vi "RT.vi"() -> ()   [LabVIEW 2023]
uses:
  <vilib>/FPGAPlugInAG/cRIO-9055/niLvFpga_Open_cRIO-9055.vi
  <vilib>/Utility/error.llb/Error Cluster From Error Code.vi
  <vilib>/rvi/errors/niLvFpgaAdjustHostInterfaceError.vi
  <vilib>/FPGAPlugInAG/cRIO-9055/niLvFpga_Run_cRIO-9055.vi
  <vilib>/FPGAPlugInAG/cRIO-9055/niLvFpga_Close_cRIO-9055.vi
  <vilib>/rvi/interface/nirviOpenFPGA/nirviOpenFPGA.xnode
  FPGA Bitfiles/projectni_FPGATarget_FPGA_GhjuFY+lihg.lvbitx
  Basic Logging/FPGA/FPGA.vi
  <vilib>/rvi/interface/nirviMethod/nirviMethod.xnode
  <vilib>/rvi/interface/nirviReadWriteControl/nirviReadWriteControl.xnode
  <vilib>/rvi/interface/nirviCloseFPGA/nirviCloseFPGA.xnode
  <vilib>/rvi/errors/niLvFpgaMergeErrorWithErrorCode.vi
  <vilib>/FPGAPlugInAG/cRIO-9055/niLvFpga_StartFifo_cRIO-9055.vi
  NiFpgaLv.dll
  <vilib>/FPGAPlugInAG/cRIO-9055/niLvFpga_ReadFifo_cRIO-9055.vi
panel:
  out "error out":errorcluster
  out "Timed Out?":bool
  out "Analog Input Chart":dbl[][](graph)
  in  "stop":bool
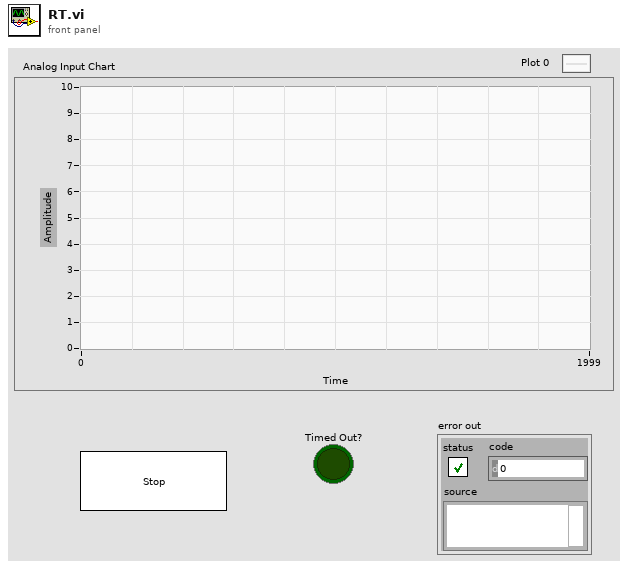
[diagram p1: front panel]
types:
  T1 = enum16{"open", "open or create", "create or replace", "create", "open (read-only)"}
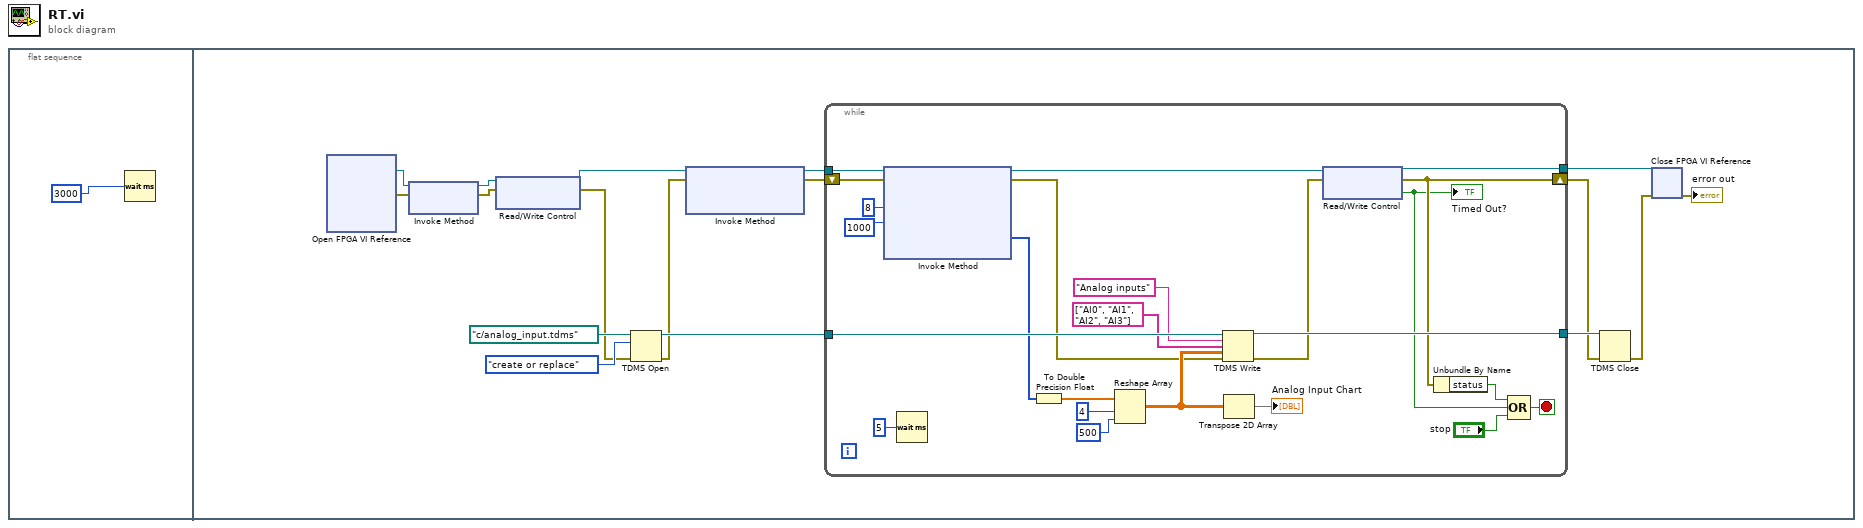
[diagram p0: block diagram]
diagram:
  n1 = flat-sequence {
    frame #0 {
      n2 = Wait (ms)(milliseconds to wait=u32 3000 ("millisecond timer value")) -> ()  [unwired: 1 out]
    }
    frame #1 {
      n3 = xnode "Open FPGA VI Reference"() -> ("FPGA VI Reference Out"=w12:refnum<k20>, "error out"=w11:errorcluster)  [unwired: 2 in]
      n4 = xnode "Invoke Method"("FPGA VI Reference In"=w12, "error in"=w11) -> ("FPGA VI Reference Out"=w5:refnum<k20>, "error out"=w4:errorcluster)
      n5 = xnode "Read/Write Control"("FPGA VI Reference In"=w5, "error in"=w4) -> ("FPGA VI Reference Out"=w3:refnum<k20>, "error out"=w2:errorcluster)  [unwired: 1 in]
      n6 = TDMS Open(8:w2, 10:T1."create or replace" ("operation (0:open)"), 11:path "c:/analog_input.tdms" ("file path")) -> (0:w9:errorcluster, 3:w16:refnum<k34>)  [unwired: 4 in]
      n7 = xnode "Invoke Method"("FPGA VI Reference In"=w3, "error in"=w9) -> ("FPGA VI Reference Out"=w18:refnum<k20>, "error out"=w13:errorcluster)  [unwired: 1 in]
      n8 = while {
        tunnel: w18 -> [w42]
        tunnel: [w32] -> w10
        tunnel: [w36] -> w17
        tunnel: w16 -> [w35]
        shift-right: [w22] -> w8
        shift-left: w13 -> [w41]
        stop <- w31 stop-if-true
        n9 = xnode "Invoke Method"("FPGA VI Reference In"=w42, "error in"=w41, "Number of Elements"=u32 8, "Timeout (ms)"=1000) -> ("FPGA VI Reference Out"=w28:refnum<k20>, "error out"=w21:errorcluster, "Data"=w27:i16[])  [unwired: 1 out]
        n10 = Wait (ms)(milliseconds to wait=u32 5) -> ()  [unwired: 1 out]
        n11 = To Double Precision Float(number=w27) -> (double precision float=w29:dbl[])
        n12 = Reshape Array(w29, 4 ("dimension size"), 500 ("dimension size")) -> (w26:dbl[][])
        n13 = TDMS Write(0:w35, 5:"Analog inputs" ("group name in (Untitled)"), 7:string[] ["AI0", "AI1", "AI2", "AI3"] ("channel name(s) in (Untitled)"), 9:w26, 11:w21) -> (4:w36:refnum<k34>, 15:w20:errorcluster)  [unwired: 1 in, 2 out]
        n14 = Transpose 2D Array(2D array=w26) -> (transposed array=→"Analog Input Chart":dbl[][])
        n15 = xnode "Read/Write Control"("FPGA VI Reference In"=w28, "error in"=w20) -> ("FPGA VI Reference Out"=w32:refnum<k20>, "error out"=w22:errorcluster, "Timed Out?"=w19:bool)
        "Timed Out?" <- w19
        n16 = Unbundle By Name(w22) -> ("status"=w25:bool)
        n17 = Compound Arithmetic op=OR(w25, w19, "stop") -> (w31:bool)
      }
      n18 = TDMS Close(8:w8, 11:w17) -> (0:w7:errorcluster)  [unwired: 1 out]
      n19 = xnode "Close FPGA VI Reference"("FPGA VI Reference In"=w10, "error in"=w7) -> ("error out"=→"error out":errorcluster)
    }
  }
